vi "Lidar Control Output Function.vi"(4 "Motor Command":fxp<+/-,18,1> format="%.18g", 6 "Lidar Motor Indicator 2":T1) -> (0 "Lidar Motor Indicator":T1, 1 "Output Voltage":fxp<+/-,20,5> format="%.17g")   [LabVIEW 2009]
uses:
  Strict Lidar Motor Indicator Cluster.ctl
  Motor Control Global.vi
  [Debug] Global.vi
panel:
  # "50Hz Update Frequency"
  # "50Hz Update Frequency"
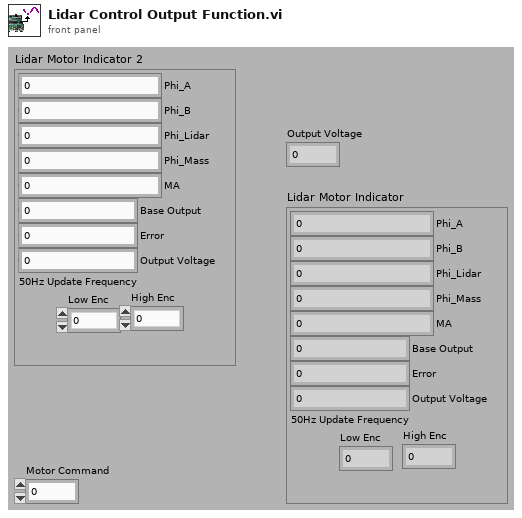
[diagram p1: front panel]
types:
  T1 = typedef "Strict Lidar Motor Indicator Cluster.ctl" = cluster{"Phi_A":fxp<+/-,18,1>, "Phi_B":fxp<+/-,18,1>, "Output Voltage":fxp<+/-,20,5>, "Phi_Lidar":fxp<+/-,18,1>, "Phi_Mass":fxp<+/-,18,1>, "MA":fxp<+/-,18,1>, "Base Output":fxp<+/-,18,1>, "Error":fxp<+/-,18,1>, "Low Enc":i32, "High Enc":i32}
  T2 = typedef "Strict Lidar Motor Control Cluster.ctl" = cluster{"Reset Encoder":bool, "Motor Enable":bool, "Choice of Control Type":enum32{"Direct Voltage Control", "Proportional Control", "PI Control", "Custom Compensator", "PID Control", "II-PID-DD Control"}, "Choice of Oscillation":enum32{"Oscillate Voltage", "Oscillate Setpoint", "No Oscillation"}, "Choice of Compensation":enum32{"None", "Computed Torque", "Mechanical Advantage", "CT & MA "}, "Choice of Error":enum32{"Gray Error", "Lidar Error", "Kent Error", "UberKent Error"}, "Units of pi rad 18b (s-fxp-1)":cluster{"Phi_B Set Point (pi rad)":fxp<+/-,18,1>, "Phi_A Set Point (pi rad)":fxp<+/-,18,1>, "Phi_Lidar Set Point (pi rad)":fxp<+/-,18,1>, "Phi_Lidar - Phi_A":fxp<+/-,18,1>, "Phi_mass-Phi_Lidar":fxp<+/-,18,1>, "Convert (enc) to (pi rad)":fxp<+/-,18,1>, "Oscillation Frequency (pi rad per 100KHz)":fxp<+/-,18,1>}, "Units of 18b (s-fxp-1) gain":cluster{"Proportional Gain":fxp<+/-,18,1>, " Integral Gain":fxp<+/-,18,1>, "Oscillation Setpoint Amplitude":fxp<+/-,18,1>, "Gravity Compensation Gain":fxp<+/-,18,1>, "Phi_B Set Point (enc) pre-gain":fxp<+/-,18,1>, "Phi_B Set Point (pi rad) pre-gain":fxp<+/-,18,1>, "Phi_A Set Point (pi rad) pre-gain":fxp<+/-,18,1>, "Phi_Lidar Set Point (pi rad) pre-gain":fxp<+/-,18,1>, "Derivative Gain":fxp<+/-,18,1>, "Double Integral Gain":fxp<+/-,18,1>, "Second Derivative Gain":fxp<+/-,18,1>}, "Units of 20b s-fxp-5 Voltage":cluster{"Oscillation Voltage Amplitude":fxp<+/-,20,5>, "Motor Voltage":fxp<+/-,20,5>}, "Units of encoder 32b uint":cluster{"Phi_B Set Point (enc)":i32, "Lidar Encoder Cap":i32}, "Debug Args":bool[], "Units of 8b int gain exponents":cluster{"Proportional Gain":i8, " Integral Gain":i8, "Oscillation Setpoint Amplitude":i8, "Gravity Compensation Gain":i8, "Phi_B Set Point (enc) pre-gain":i8, "Phi_B Set Point (pi rad) pre-gain":i8, "Phi_A Set Point (pi rad) pre-gain":i8, "Phi_Lidar Set Point (pi rad) pre-gain":i8, "Derivative Gain":i8, "Double Integral Gain":i8, "Second Derivative Gain":i8}, "6b (u-fxp-6)":cluster{"Size of Integrator":fxp<+,6,6>, "Size of IIntigrator":fxp<+,6,6>, "Size of Differentiator":fxp<+,6,6>, "Size of DDifferentiator":fxp<+,6,6>}}
  T3 = enum32{"Direct Voltage Control", "Proportional Control", "PI Control", "Custom Compensator", "PID Control", "II-PID-DD Control"}
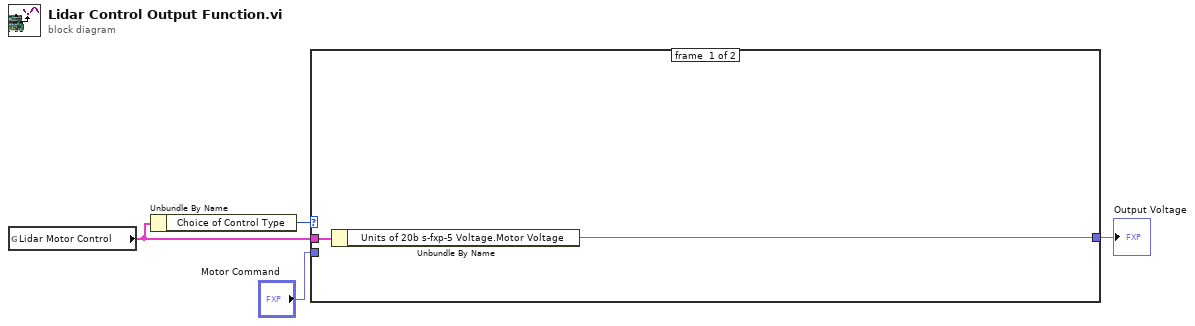
[diagram p0: block diagram]
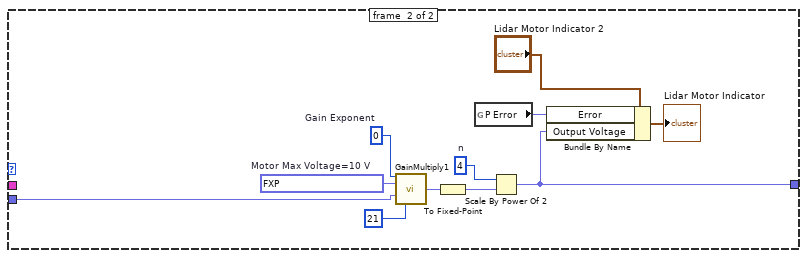
[diagram p2: hidden frame]
diagram:
  n1 = global read "Motor Control Global.vi" "Lidar Motor Control"() -> (w1:T2)
  n2 = Unbundle By Name(w1) -> ("Choice of Control Type"=w2:T3)
  n3 = case shown="Default" w2 {
    tunnel: "Motor Command" -> [_ w13]
    tunnel: [w5 w10] -> w3
    tunnel: w1 -> [w6 _]
    frame #0 {
      n4 = Unbundle By Name(w6) -> ("Units of 20b s-fxp-5 Voltage.Motor Voltage"=w5:fxp<+/-,20,5>)
    }
    frame #1 {
      w15 = i8 0  # Gain Exponent
      w12 = 4  # n
      w14 = fxp<+/-,18,1> 0.625  # Motor Max Voltage=10 V
      n5 = call "GainMultiply1.vi"("Gain Exponent"=w15, "Gain"=w14, "Input"=w13, "Unique 8b identifier"=u8 21) -> ("Output"=w17:fxp<+/-,18,1>)  [unwired: 9 in, 2 out]
      n6 = To Fixed-Point(number=w17) -> (fixed-point=w11:fxp<+/-,20,5>)  [unwired: 1 in]
      n7 = global read "[Debug] Global.vi" "P Error"() -> (w7:fxp<+/-,18,1>)
      n8 = Scale By Power Of 2(n=w12, x=w11) -> (x*2^n=w10:fxp<+/-,20,5>)
      n9 = Bundle By Name(cluster="Lidar Motor Indicator 2", "Error"=w7, "Output Voltage"=w10) -> (→"Lidar Motor Indicator":T1)
    }
  }
  "Output Voltage" <- w3
